vi "Main Page.vi"(8 "error in (no error)":errorcluster, 11 "Node Ptr":T2 format="%.0x") -> (0 "error out":errorcluster)   [LabVIEW 2024, in "Embedded TDMS Logger System Explorer.lvlib"]
doc: "The UI Page giving the user the ability to modify properties on the file level of the custom device, i.e.:\n- Segmentation options\n- Meta Data to be logged on the file level of the TDMS\n- Naming convention of the file\n- Name of the Custom Device\n- Directory to log files into."
uses:
  Embedded TDMS Logger System Explorer.lvlib
  <vilib>/NI VeriStand/Custom Device API/Custom Device Item Ref.ctl
  Shared/SegmentOptions.ctl
  <vilib>/NI VeriStand/Custom Device API/Get Item Property (U16).vi
  <vilib>/NI VeriStand/Custom Device API/Get Item Property (Variant).vi
  <vilib>/NI VeriStand/Custom Device API/Set Item Property (Variant).vi
  <vilib>/NI VeriStand/Custom Device API/Set Item Property (U16).vi
  <vilib>/NI VeriStand/Custom Device API/Set Item Property (String).vi
  <vilib>/NI VeriStand/Custom Device API/Set Item Property (Boolean).vi
  <vilib>/NI VeriStand/Custom Device API/Set Item Property (U64).vi
  <vilib>/NI VeriStand/Custom Device API/Custom Device API.lvlib
  Shared/File Classes/Meta Data.ctl
panel:
  in  "Tab Control":enum32{"File Settings", "Meta Data"}(tab)
  out "String 3":string="The data format can be specified in the string, as with the formats specified in: https://www.ni.com/docs/en-US/bundle/labview-api-ref/page/functions/format-date-time-string.html"
  in  "Segment every":dbl=3600.0
  in  "Segment by":T1=enum."Size (MB)"
  in  "Filename Format:":string="mytestfile_%Y-%m-%d-%H-%M-%S.tdms"
  in  "Log Directory":string
  in  "Segment Files":bool=TRUE
  in  "File Level Meta Data":string[][](table)=[["Software Version"], ["Test Rig Used"], ["UUT"], ["Operator"]]
  in  "Async Timeout (ms)":u16
  out "Version":string
  in  "Specific Header":cluster{"Section Name":string}={"Section Name"="Custom Device Item Settings"}
  in  "General Header":cluster{"Section Name":string}={"Section Name"="General Custom Device Settings"}
  in  "Description":string
  in  "Name":string
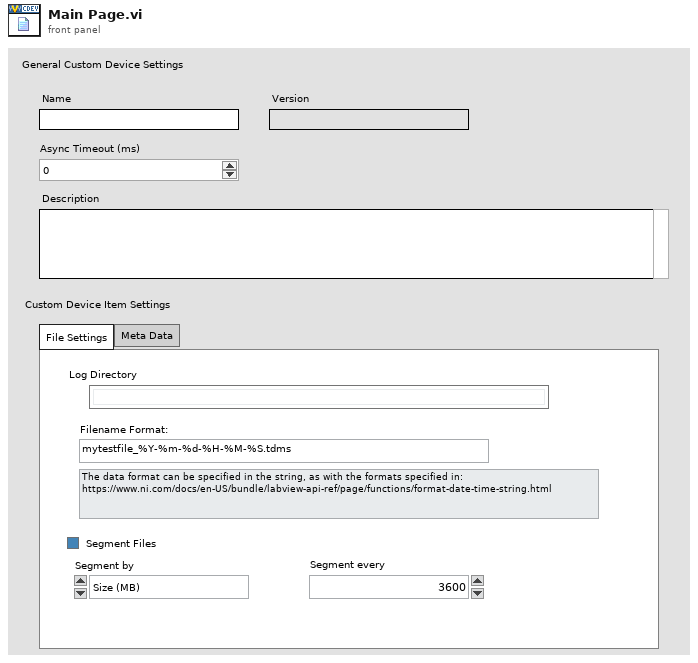
[diagram p1: front panel]
types:
  T1 = typedef "SegmentOptions.ctl" = enum16{"Time (s)", "Size (MB)"}
  T2 = typedef "Custom Device API.lvlib/Custom Device Item Ref.ctl" = u64
  T3 = typedef "Custom Device API.lvlib/Custom Device Item Info.ctl" = cluster{"Name":string, "Is Channel":bool, "GUID":string, "Is Waveform":bool}
  T4 = typedef "Meta Data.ctl" = cluster{"Key":string, "Value":string}
  T5 = typedef "Custom Device API.lvlib/Custom Device Commands.ctl" = enum16{"Default", "Item renamed", "Shutdown", "Dynamic button pressed"}
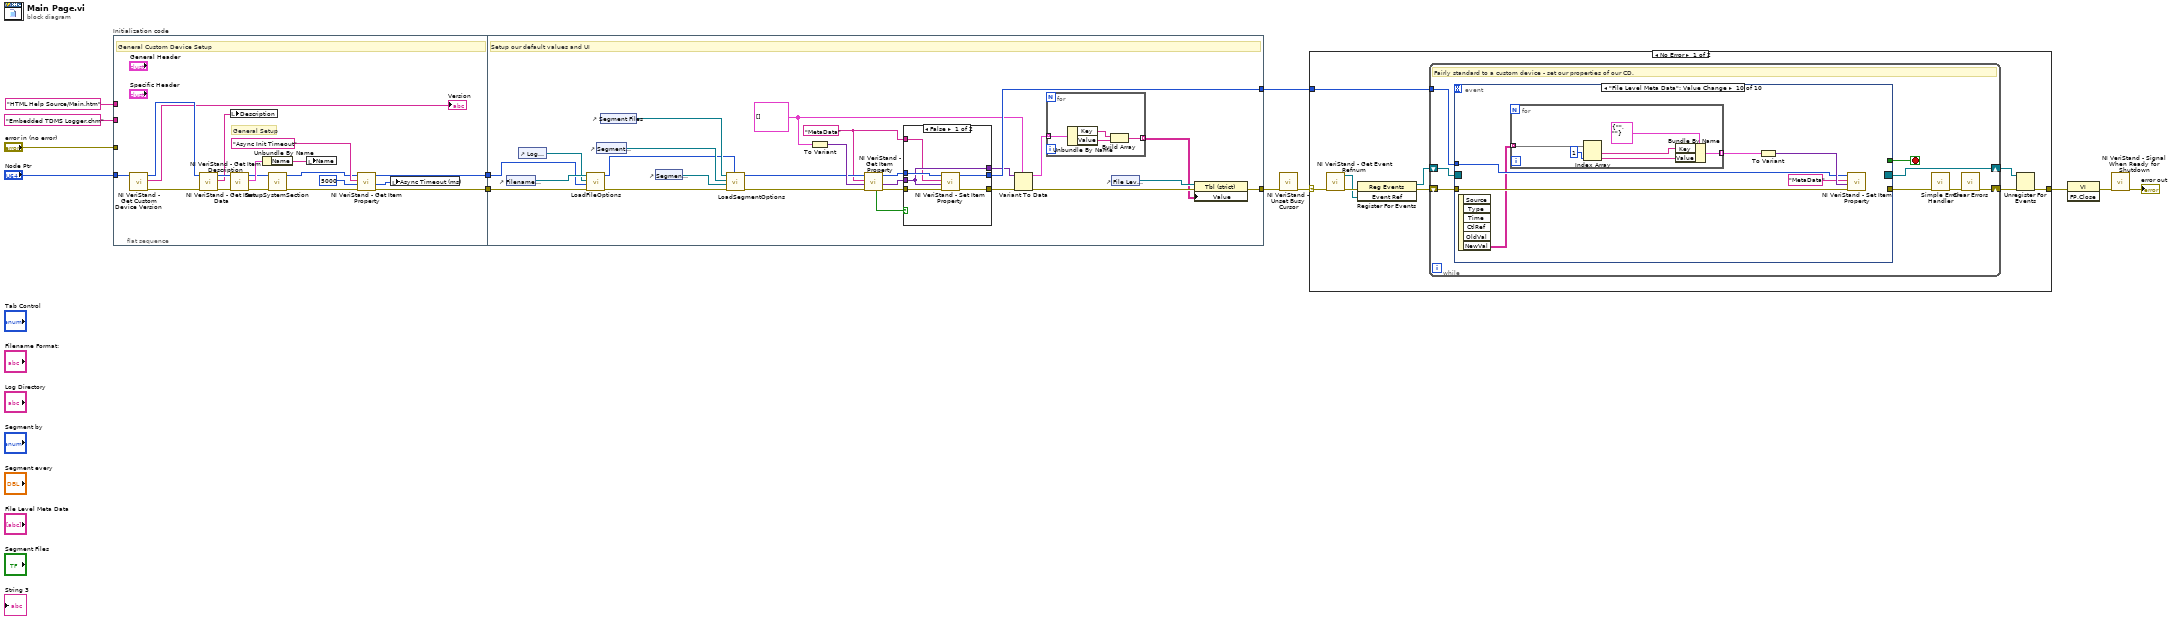
[diagram p0: block diagram]
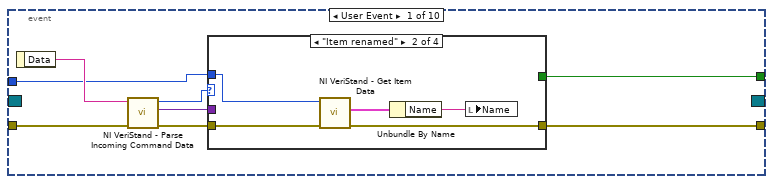
[diagram p2: hidden frame]
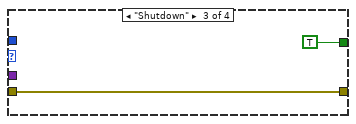
[diagram p4: hidden frame]
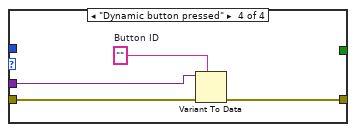
[diagram p5: hidden frame]
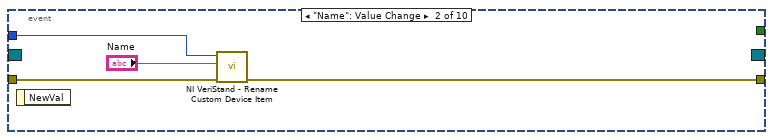
[diagram p6: hidden frame]
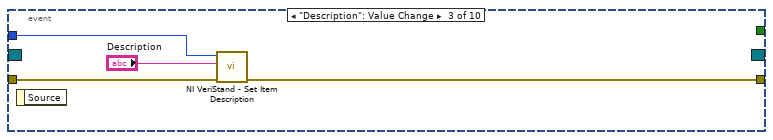
[diagram p7: hidden frame]
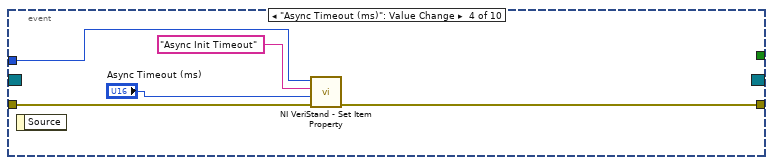
[diagram p8: hidden frame]
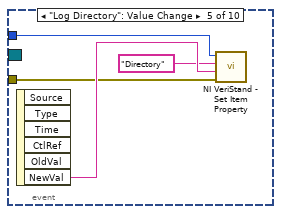
[diagram p9: hidden frame]
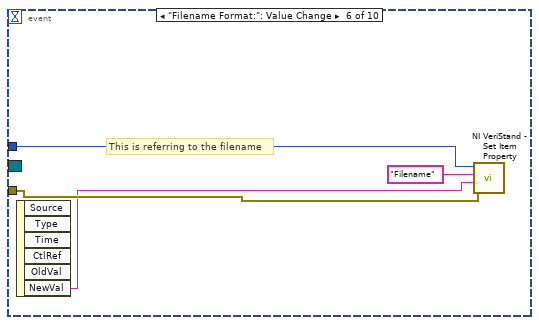
[diagram p10: hidden frame]
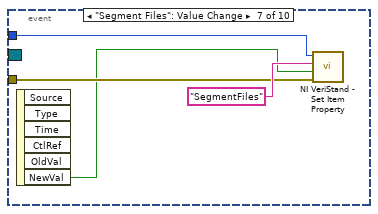
[diagram p11: hidden frame]
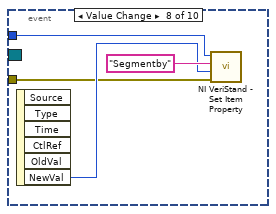
[diagram p12: hidden frame]
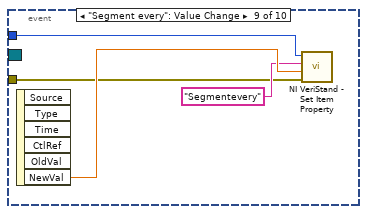
[diagram p13: hidden frame]
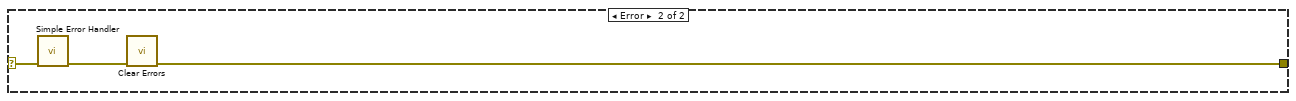
[diagram p14: hidden frame]
diagram:
  n1 = flat-sequence "Initialization code" {
    tunnel: "error in (no error)" -> [_]
    tunnel: "Node Ptr" -> [w27]
    tunnel: "HTML Help Source/Main.htm" ("HTML File") -> [_]
    tunnel: "Embedded TDMS Logger.chm" ("CD_CHM_FileName") -> [_]
    tunnel: [w18] -> w4
    tunnel: [w17] -> w3
    tunnel: w4 -> [w56]
    tunnel: w3 -> [w31]
    tunnel: [w43] -> w2
    tunnel: [w42] -> w1
    frame #0 {
      # "General Setup"
      # "General Custom Device Setup"
      n2 = call <vilib>:"NI VeriStand - Get Custom Device Version.vi"("Device Ref in"=w27) -> ("error out"=w26:errorcluster, "Value"=→"Version":string, "Device Ref out"=w25:T2)  [unwired: 8 in]
      n3 = call <vilib>:"NI VeriStand - Get Item Description.vi"("error in (no error)"=w26, "Item Ref in"=w25) -> ("error out"=w29:errorcluster, "Description"=w22:string, "Item Ref out"=w30:T2)  [unwired: 7 out]
      n4 = local write "Description"(w22) -> ()
      n5 = call <vilib>:"NI VeriStand - Get Item Data.vi"("error in (no error)"=w29, "Item Ref in"=w30) -> ("error out"=w15:errorcluster, "Item Info"=w28:T3, "Item Ref out"=w16:T2)  [unwired: 7 out]
      n6 = Unbundle By Name(w28) -> ("Name"=w23:string)
      n7 = call "SetupSystemSection.vi"("error in (no error)"=w15, "Node Ptr"=w16) -> ("error out"=w14:errorcluster, "Parent Ref Out"=w13:T2)  [unwired: 5 in, 3 out]
      n8 = local write "Name"(w23) -> ()
      n9 = call-poly <vilib>:"NI VeriStand - Get Item Property.vi"("error in (no error)"=w14, "Default Value"=u16 5000, "Property Name"="Async Init Timeout", "Item Ref in"=w13) -> ("error out"=w18:errorcluster, "Value"=w21:u16, "Item Ref out"=w17:T2)  [unwired: 4 in, 1 out]
      n10 = local write "Async Timeout (ms)"(w21) -> ()
    }
    frame #1 {
      w33 = T4[] []
      w40 = "MetaData" ("Property Name")
      # "Setup our default values and UI"
      n11 = control-ref of="Filename Format:"() -> (w55:refnum<vi>)
      n12 = control-ref of="Log Directory"() -> (w32:refnum<vi>)
      n13 = call "LoadFileOptions.vi"("error in (no error)"=w56, "Item Ref in"=w31, "Directory In"=w32, "Filename in"=w55) -> ("error out"=w54:errorcluster, "Item Ref out"=w51:T2)  [unwired: 6 in]
      n14 = control-ref of="Segment every"() -> (w53:refnum<vi>)
      n15 = control-ref of="Segment Files"() -> (w52:refnum<vi>)
      n16 = control-ref of="Segment by"() -> (w50:refnum<vi>)
      n17 = call "LoadSegmentOptions.vi"("Item Ref in"=w51, "error in (no error)"=w54, "Segment by"=w50, "Segment every"=w53, "Boolean in"=w52) -> ("error out"=w41:errorcluster, "Item Ref out"=w45:T2)  [unwired: 5 in]
      n18 = To Variant(anything=w33) -> (Variant=w46:variant)
      n19 = call-poly <vilib>:"NI VeriStand - Get Item Property.vi"("error in (no error)"=w41, "Default Value"=w46, "Property Name"=w40, "Item Ref in"=w45) -> ("error out"=w48:errorcluster, "Value"=w47:variant, "Item Ref out"=w44:T2, "Found?"=w49:bool)  [unwired: 4 in]
      n20 = case shown="False" w49 {
        tunnel: [w66 w69] -> w43
        tunnel: w44 -> [w65 w69]
        tunnel: [w64 w68] -> w38
        tunnel: w48 -> [w63 w68]
        tunnel: w47 -> [w62 w67]
        tunnel: [w62 w67] -> w36
        tunnel: w40 -> [w61 _]
        frame False {
          n21 = call-poly <vilib>:"NI VeriStand - Set Item Property.vi"("error in (no error)"=w63, "Value"=w62, "Property Name"=w61, "Item Ref in"=w65) -> ("error out"=w64:errorcluster, "Item Ref out"=w66:T2)  [unwired: 5 in, 1 out]
        }
        frame True {
        }
      }
      n22 = Variant To Data(error in=w38, type=w33, Variant=w36) -> (data=w34:T4[], error out=w37:errorcluster)
      n23 = for {
        tunnel: [w58] -> w35 mode=indexing
        tunnel: w34 -> [w57] mode=indexing
        n24 = Unbundle By Name(w57) -> ("Key"=w60:string, "Value"=w59:string)
        n25 = Build Array(w60, w59) -> (w58:string[])
      }
      n26 = control-ref of="File Level Meta Data"() -> (w39:refnum<vi>)
      n27 = property class="Tbl (strict)"(reference=w39, error in=w37, "Value"=w35) -> (error out=w42:errorcluster)  [unwired: 1 out]
    }
  }
  n28 = call <vilib>:"NI VeriStand - Unset Busy Cursor.vi"("error in (no error)"=w1) -> ("error out"=w8:errorcluster)  [unwired: 10 out]
  n29 = case shown="No Error" w8 {
    selector: w8 -> [w71 w154]
    tunnel: [w75 w152] -> w12
    tunnel: w2 -> [w70 _]
    frame No Error {
      n30 = call <vilib>:"NI VeriStand - Get Event Refnum.vi"("error in (no error)"=w71) -> ("error out"=w78:errorcluster, "Event Ref"=w74:refnum<user-event>)  [unwired: 9 out]
      n31 = register-events(error in=w78, w74) -> (reference out=w72:refnum<event-registration>, error out=w73:errorcluster)  [unwired: 1 in]
      n32 = while {
        shift-right: [w80] -> w76
        shift-left: w73 -> [w85]
        shift-right: [w86] -> w77
        shift-left: w72 -> [w84]
        tunnel: w70 -> [w79]
        stop <- w83 stop-if-true
        # "Fairly standard to a custom device - set our properties of our CD."
        n33 = event shown="[9] \"File Level Meta Data\": Value Change" {
          selector: w84 -> [_ _ _ _ _ _ _ _ _ _]
          dyn-events: [_ _ _ _ _ _ _ _ _ _] -> w86
          timeout: _ -> [_ _ _ _ _ _ _ _ _ _]
          tunnel: w85 -> [w94 w110 w114 w119 w121 w126 w130 w132 w136 w142]
          tunnel: [w90 _ _ _ _ _ _ _ _ _] -> w83
          tunnel: [w89 w109 w113 w117 _ _ _ _ _ _] -> w82
          tunnel: w79 -> [w87 w107 w111 w115 w120 w124 w129 w133 w138 w143]
          event User Event {
            n34 = event-data() -> ("Data"=w93:string)  [unwired: 1 out]
            n35 = call <vilib>:"NI VeriStand - Parse Incoming Command Data.vi"("error in (no error)"=w94, "Incoming data"=w93) -> ("error out"=w92:errorcluster, "Outgoing data"=w88:variant, "Action"=w91:T5)  [unwired: 7 out]
            n36 = case shown="\"Item renamed\"" w91 {
              tunnel: w92 -> [w95 w100 w101 w106]
              tunnel: [_ _ TRUE _] -> w90
              tunnel: [w95 w98 w101 w103] -> w89
              tunnel: w88 -> [_ _ _ w105]
              tunnel: w87 -> [_ w96 _ _]
              frame "Default", Default {
              }
              frame "Item renamed" {
                n37 = call <vilib>:"NI VeriStand - Get Item Data.vi"("error in (no error)"=w100, "Item Ref in"=w96) -> ("error out"=w98:errorcluster, "Item Info"=w99:T3)  [unwired: 8 out]
                n38 = Unbundle By Name(w99) -> ("Name"=w97:string)
                n39 = local write "Name"(w97) -> ()
              }
              frame "Shutdown" {
              }
              frame "Dynamic button pressed" {
                w104 = ""  # Button ID
                n40 = Variant To Data(error in=w106, type=w104, Variant=w105) -> (error out=w103:errorcluster)  [unwired: 1 out]
              }
            }
          }
          event "Name": Value Change {
            n41 = event-data() -> ()  [unwired: 2 out]
            n42 = call <vilib>:"NI VeriStand - Rename Custom Device Item.vi"("error in (no error)"=w110, "New Name"="Name", "Item Ref in"=w107) -> ("error out"=w109:errorcluster)  [unwired: 1 in, 7 out]
          }
          event "Description": Value Change {
            n43 = event-data() -> ()  [unwired: 2 out]
            n44 = call <vilib>:"NI VeriStand - Set Item Description.vi"("error in (no error)"=w114, "Description"="Description", "Item Ref in"=w111) -> ("error out"=w113:errorcluster)  [unwired: 8 out]
          }
          event "Async Timeout (ms)": Value Change {
            n45 = event-data() -> ()  [unwired: 2 out]
            n46 = call-poly <vilib>:"NI VeriStand - Set Item Property.vi"("error in (no error)"=w119, "Value"="Async Timeout (ms)", "Property Name"="Async Init Timeout", "Item Ref in"=w115) -> ("error out"=w117:errorcluster)  [unwired: 5 in, 2 out]
          }
          event "Log Directory": Value Change {
            n47 = event-data() -> ("NewVal"=w123:string)  [unwired: 6 out]
            n48 = call-poly <vilib>:"NI VeriStand - Set Item Property.vi"("error in (no error)"=w121, "Value"=w123, "Property Name"="Directory", "Item Ref in"=w120) -> ()  [unwired: 5 in, 3 out]
          }
          event "Filename Format:": Value Change {
            # "This is referring to the filename"
            n49 = event-data() -> ("NewVal"=w125:string)  [unwired: 6 out]
            n50 = call-poly <vilib>:"NI VeriStand - Set Item Property.vi"("error in (no error)"=w126, "Value"=w125, "Property Name"="Filename", "Item Ref in"=w124) -> ()  [unwired: 5 in, 3 out]
          }
          event "Segment Files": Value Change {
            n51 = event-data() -> ("NewVal"=w128:bool)  [unwired: 6 out]
            n52 = call-poly <vilib>:"NI VeriStand - Set Item Property.vi"("error in (no error)"=w130, "Value"=w128, "Property Name"="SegmentFiles", "Item Ref in"=w129) -> ()  [unwired: 5 in, 3 out]
          }
          event Value Change {
            n53 = event-data() -> ("NewVal"=w134:T1)  [unwired: 6 out]
            n54 = call-poly <vilib>:"NI VeriStand - Set Item Property.vi"("error in (no error)"=w132, "Value"=w134, "Property Name"="Segmentby", "Item Ref in"=w133) -> ()  [unwired: 5 in, 3 out]
          }
          event "Segment every": Value Change {
            n55 = event-data() -> ("NewVal"=w139:dbl)  [unwired: 6 out]
            n56 = call-poly <vilib>:"NI VeriStand - Set Item Property.vi"("error in (no error)"=w136, "Value"=w139, "Property Name"="Segmentevery", "Item Ref in"=w138) -> ()  [unwired: 5 in, 3 out]
          }
          event "File Level Meta Data": Value Change {
            n57 = event-data() -> ("NewVal"=w140:string[][])  [unwired: 6 out]
            n58 = for {
              tunnel: [w151] -> w141 mode=indexing
              tunnel: w140 -> [w147] mode=indexing
              n59 = Index Array(array=w147, index #2=1 ("index")) -> (element #1=w148:string, element #2=w149:string)  [unwired: 1 in]
              n60 = Bundle By Name(cluster=T4 {"Key"="", "Value"=""} ("Meta Data"), "Key"=w148, "Value"=w149) -> (w151:T4)
            }
            n61 = To Variant(anything=w141) -> (Variant=w145:variant)
            n62 = call-poly <vilib>:"NI VeriStand - Set Item Property.vi"("error in (no error)"=w142, "Value"=w145, "Property Name"="MetaData", "Item Ref in"=w143) -> ()  [unwired: 5 in, 3 out]
          }
        }
        n63 = call <vilib>:"Simple Error Handler.vi"("error in (no error)"=w82) -> ("error out"=w81:errorcluster)  [unwired: 1 in, 7 out]
        n64 = call <vilib>:"Clear Errors.vi"("error in (no error)"=w81) -> ("error out"=w80:errorcluster)  [unwired: 1 in, 5 out]
      }
      n65 = Unregister For Events(event registration refnum=w77, error in=w76) -> (error out=w75:errorcluster)
    }
    frame Error {
      n66 = call <vilib>:"Simple Error Handler.vi"("error in (no error)"=w154) -> ("error out"=w153:errorcluster)  [unwired: 1 in, 7 out]
      n67 = call <vilib>:"Clear Errors.vi"("error in (no error)"=w153) -> ("error out"=w152:errorcluster)  [unwired: 1 in, 5 out]
    }
  }
  n68 = invoke class="VI" method="FP.Close"(error in=w12) -> (error out=w11:errorcluster)  [unwired: 2 in, 2 out]
  n69 = call <vilib>:"NI VeriStand - Signal When Ready for Shutdown.vi"("error in (no error)"=w11) -> ("error out"=→"error out":errorcluster)  [unwired: 10 out]
